vi "ReadData_8532.vi"(8 "error in (no error)":errorcluster, 9 "pDMAStatus":i32[](array[numeric]), 10 "Buffer":u16[](array[numeric]), 11 "task":T1={"Task Info"={"Accele Task"=[], "Simulate"=FALSE, "采样率"={"AISampleRate"=10123, "CouplingType"=10000, "Butter"=1000}, "Trig"={"PreTrigCNT"=0, "TriggerMode"=enum."中间触发", "TriggerSource"=enum."软件触发", "ATRTriggerChannel"=enum."通道0", "TriggerDir"=enum."下降沿触发", "TrigLevelVolt"=0.0, "bAvailableTrig"=FALSE}, "clock"={"EN"=FALSE, "clocksource"=enum."内部时钟", "outclocksource"=enum."Trig0"}, "delay(S)"=0.0}, "datain"={"nSegmentCount"=0, "chaneldataSize"=8192, "t0 in"=timestamp(0 s since 1904-01-01), "nsegmentsize"=0, "chanelcouter"=0}, "times"=0.0, "timer"=[], "\nen"=FALSE} {"Task Info"."采样率"."CouplingType" items=["直流耦合", "交流耦合"]}) -> (0 "error out":errorcluster, 1 "pDMAStatus out":i32[](array[numeric]), 2 "Data":waveform(dbl)[](array[waveform]), 3 "task out":T1={"Task Info"={"Accele Task"=[], "Simulate"=FALSE, "采样率"={"AISampleRate"=10123, "CouplingType"=10000, "Butter"=1000}, "Trig"={"PreTrigCNT"=0, "TriggerMode"=enum."中间触发", "TriggerSource"=enum."软件触发", "ATRTriggerChannel"=enum."通道0", "TriggerDir"=enum."下降沿触发", "TrigLevelVolt"=0.0, "bAvailableTrig"=FALSE}, "clock"={"EN"=FALSE, "clocksource"=enum."内部时钟", "outclocksource"=enum."Trig0"}, "delay(S)"=0.0}, "datain"={"nSegmentCount"=0, "chaneldataSize"=8192, "t0 in"=timestamp(0 s since 1904-01-01), "nsegmentsize"=0, "chanelcouter"=0}, "times"=0.0, "timer"=[], "\nen"=FALSE} {"Task Info"."采样率"."CouplingType" items=["直流耦合", "交流耦合"]})   [LabVIEW 2009]
uses:
  Data.vi
  PCI8532_32.dll
  Ctrls/Acceleration Channel Config_Ctrls-某型振动实验台测试系统.ctl
  Ctrls/Sample Information.ctl
  Ctrls/Trig.ctl
  Ctrls/clock.ctl
  Ctrls/Task Info.ctl
  Ctrls/DATA info.ctl
  Ctrls/task.ctl
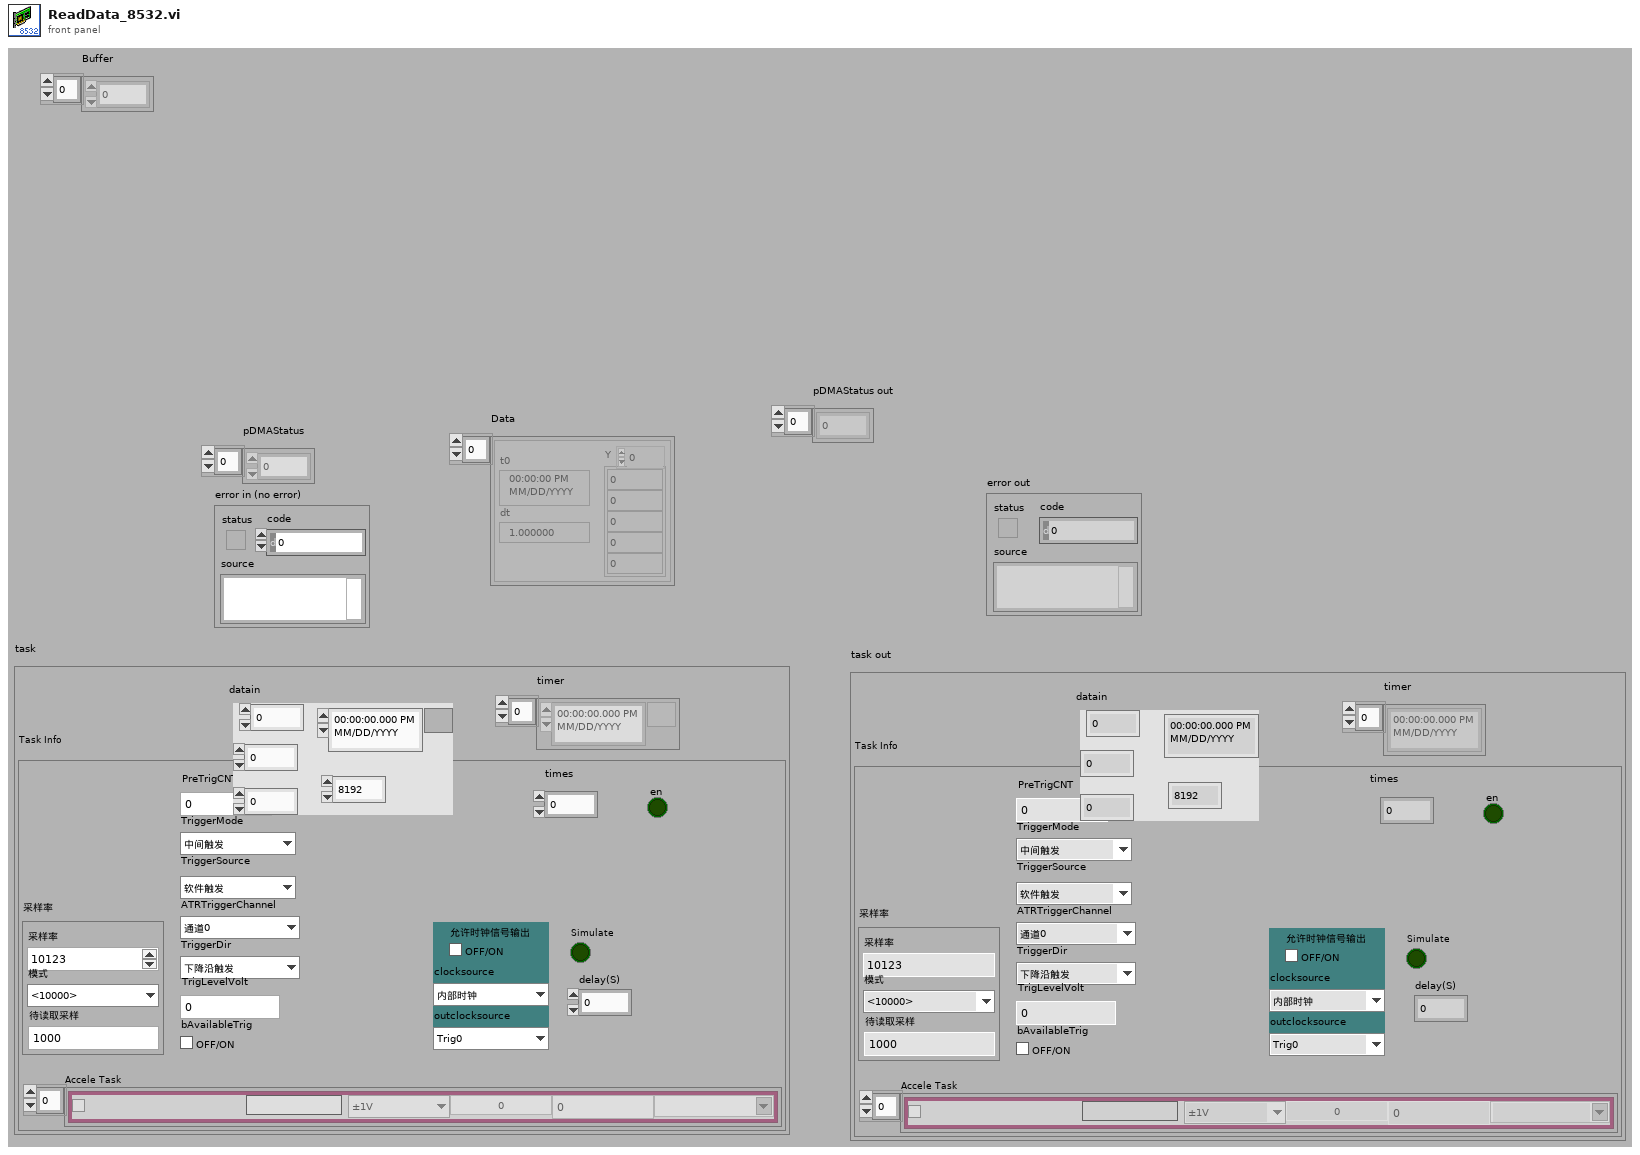
[diagram p1: front panel]
types:
  T1 = typedef "task.ctl" = cluster{"Task Info":T2, "datain":T7, "times":dbl, "timer":timestamp[], "\nen":bool}
  T2 = typedef "Task Info.ctl" = cluster{"Accele Task":T3[], "Simulate":bool, "采样率":T4, "Trig":T5, "clock":T6, "delay(S)":dbl}
  T3 = typedef "Acceleration Channel Config_Ctrls-某型振动实验台测试系统.ctl" = cluster{"Enable":bool, "Name":string, "range":enum16{"±1V", "±5V"}, "SensValue":dbl, "PhysicalName":string, "off":dbl, "Sensunits":string}
  T4 = typedef "Sample Information.ctl" = cluster{"AISampleRate":i32, "CouplingType":i32, "Butter":i32}
  T5 = typedef "Trig.ctl" = cluster{"PreTrigCNT":i32, "TriggerMode":enum16{"中间触发", "后触发", "预触发", "硬件延时触发"}, "TriggerSource":enum16{"软件触发", "DTR信号源", "ATR信号源", "Triger信号触发"}, "ATRTriggerChannel":enum16{"通道0", "通道1", "通道2", "通道3"}, "TriggerDir":enum16{"下降沿触发", "上升沿触发", "上下边没均触发"}, "TrigLevelVolt":sgl, "bAvailableTrig":bool}
  T6 = typedef "clock.ctl" = cluster{"EN":bool, "clocksource":enum16{"内部时钟", "外部时钟"}, "outclocksource":enum16{"Trig0", "Trig1", "Trig2", "Trig3", "Trig4", "Trig5", "Trig6", "Trig7", "PXI_STAR"}}
  T7 = typedef "DATA info.ctl" = cluster{"nSegmentCount":i32, "chaneldataSize":i32, "t0 in":timestamp, "nsegmentsize":i32, "chanelcouter":i32}
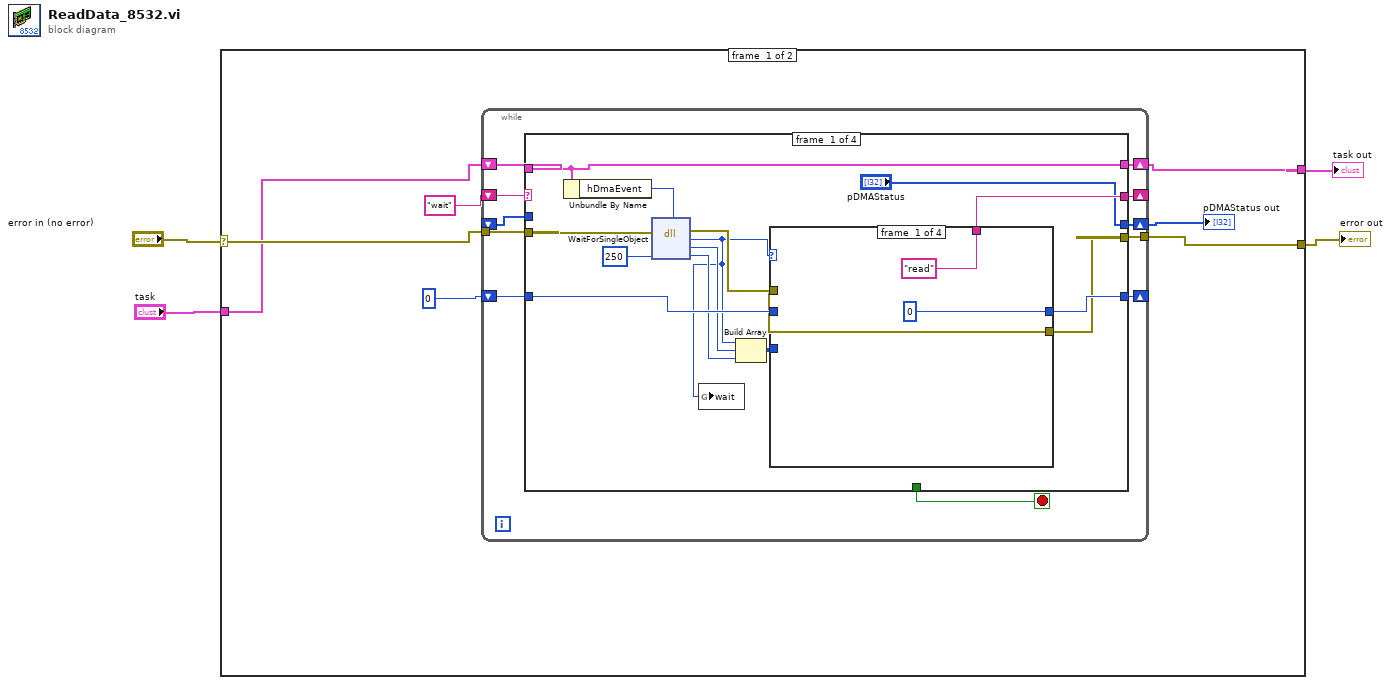
[diagram p0: block diagram]
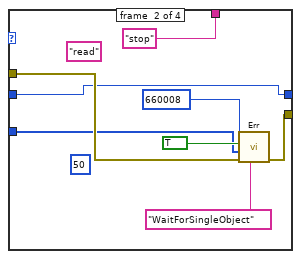
[diagram p2: hidden frame]
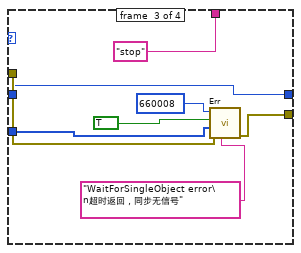
[diagram p3: hidden frame]
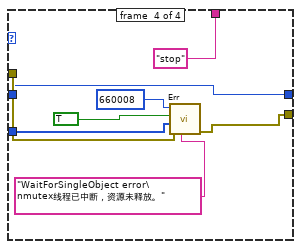
[diagram p4: hidden frame]
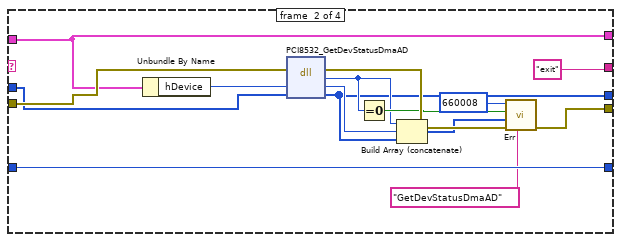
[diagram p5: hidden frame]
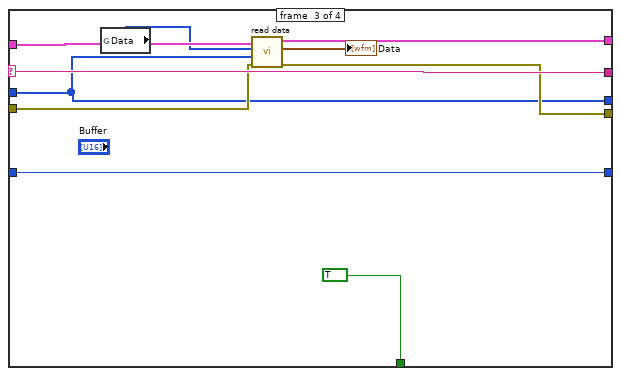
[diagram p6: hidden frame]
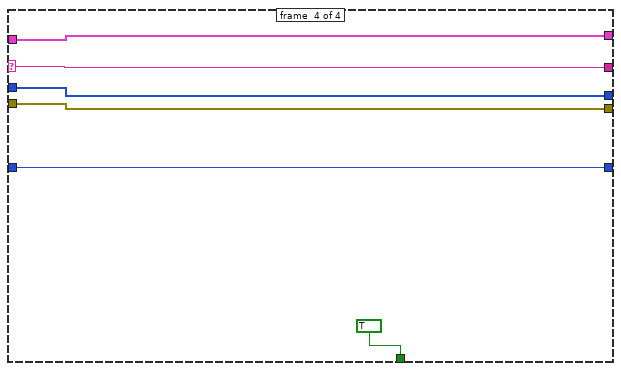
[diagram p7: hidden frame]
diagram:
  n1 = case shown="无错误" "error in (no error)" {
    selector: "error in (no error)" -> [w10 w96]
    tunnel: [w11 w96] -> w4
    tunnel: "task" -> [w9 w95]
    tunnel: [w8 w95] -> w1
    frame #0 {
      n2 = while {
        shift-right: [w19] -> _
        shift-left: "wait" -> [w22]
        tunnel: w10 -> [w20]
        tunnel: [w18] -> w11
        shift-right: [w17] -> _
        shift-left: 0 -> [w16]
        shift-right: [w14] -> w5
        shift-left: _ -> [w13]
        shift-right: [w12] -> w8
        shift-left: w9 -> [w21]
        stop <- w15 stop-if-true
        n3 = case shown="\"exit\"" w22 {
          selector: w22 -> [_ _ w86 w92]
          tunnel: [w29 w73 w82 w89] -> w18
          tunnel: w21 -> [w28 w74 w85 w91]
          tunnel: w20 -> [w34 w77 w84 w89]
          tunnel: [w33 "exit" ("t") w86 w92] -> w19
          tunnel: w16 -> [w32 w78 w87 w93]
          tunnel: [w31 w78 w87 w93] -> w17
          tunnel: [_ _ TRUE TRUE] -> w15
          tunnel: ["pDMAStatus" w66 w80 w90] -> w14
          tunnel: w13 -> [_ w64 w80 w90]
          tunnel: [w28 w74 w83 w91] -> w12
          frame #0 {
            n4 = Unbundle By Name(w28) -> ("hDmaEvent"=w35:i32)
            n5 = dll-call lib="kernel32" fn="WaitForSingleObject"(error in=w34, "hEvent"=w35, "dwMilliseconds"=250 ("millisecond multiple")) -> (error out=w30:errorcluster, w24:u32, "hEvent"=w27:i32, "dwMilliseconds"=w26:i32)  [unwired: 2 in, 1 out]
            n6 = global write "Data.vi" "wait"(w24) -> ()
            n7 = Build Array(w24, w27, w26) -> (w25:u32[])
            n8 = case shown="258" w24 {
              tunnel: ["read" "stop" ("t") "stop" ("t") "stop" ("t")] -> w33
              tunnel: w32 -> [_ w41 w49 w56]
              tunnel: [0 w41 w49 w56] -> w31
              tunnel: w30 -> [w37 w43 w51 w58]
              tunnel: [w37 w44 w52 w63] -> w29
              tunnel: w25 -> [_ w42 w50 w60]
              frame #0 {
              }
              frame #1 {
                (unwired) "read"
                (unwired) u32 50 ("millisecond multiple")
                n9 = call "Err.vi"("source"="WaitForSingleObject", "error in (no error)"=w43, "Par"=w42, "error?"=TRUE, "code"=660008) -> ("error out"=w44:errorcluster)  [unwired: 6 out]
              }
              frame #2 {
                n10 = call "Err.vi"("source"="WaitForSingleObject error\n超时返回，同步无信号", "error in (no error)"=w51, "Par"=w50, "error?"=TRUE, "code"=660008) -> ("error out"=w52:errorcluster)  [unwired: 6 out]
              }
              frame #3 {
                n11 = call "Err.vi"("source"="WaitForSingleObject error\nmutex线程已中断，资源未释放。", "error in (no error)"=w58, "Par"=w60, "error?"=TRUE, "code"=660008) -> ("error out"=w63:errorcluster)  [unwired: 6 out]
              }
            }
          }
          frame #1 {
            n12 = Unbundle By Name(w74) -> ("hDevice"=w76:i32)
            n13 = dll-call lib="PCI8532_32.dll" fn="PCI8532_GetDevStatusDmaAD" label="GetDevStatusDmaAD"(error in=w77, "hDevice"=w76, "pDMAStatus"=w64) -> (error out=w72:errorcluster, "返回类型"=w68:i32, "hDevice"=w67:i32, "pDMAStatus"=w66:i32[])  [unwired: 2 in, 1 out]
            n14 = Equal To 0?(x=w68) -> (x = 0?=w71:bool)
            n15 = Build Array (concatenate)(w68, w67, w66) -> (w69:i32[])
            n16 = call "Err.vi"("source"="GetDevStatusDmaAD", "error in (no error)"=w72, "Par"=w69, "error?"=w71, "code"=660008) -> ("error out"=w73:errorcluster)  [unwired: 6 out]
          }
          frame #2 {
            n17 = global read "Data.vi" "Data"() -> (w79:u16[])
            n18 = call "read data.vi"("error in (no error)"=w84, "pDMAStatus"=w80, "Buffer"=w79, "task"=w85) -> ("error out"=w82:errorcluster, "Data"=→"Data":waveform(dbl)[], "task out"=w83:T1)  [unwired: 5 out]
          }
          frame #3 {
          }
        }
      }
      "pDMAStatus out" <- w5
    }
    frame #1 {
    }
  }
  "error out" <- w4
  "task out" <- w1
